vi "Blacklist Channel.vi"(8 "error in (no error)":errorcluster, 9 "Channel 2":string, 10 "Channel 1":string, 11 "SLSC Switch in":refnum<class "SLSC Switch.lvclass">) -> (0 "error out":errorcluster, 1 "New Entry?":bool, 3 "SLSC Switch out":refnum<class "SLSC Switch.lvclass">)   [LabVIEW 2015, in "SLSC Switch.lvclass"]
uses:
  SLSC Switch.lvclass
  SLSC Switch.lvclass/SLSC Switch.ctl
  Controls/Connection.ctl
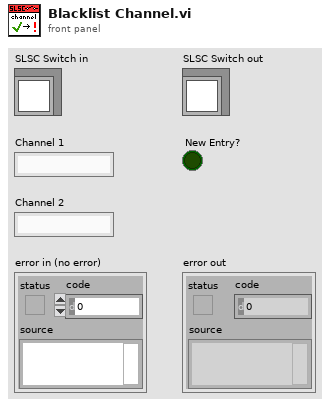
[diagram p1: front panel]
types:
  T1 = typedef "SLSC Switch.lvclass/Connection.ctl" = cluster{"channel 1":string, "channel 2":string}
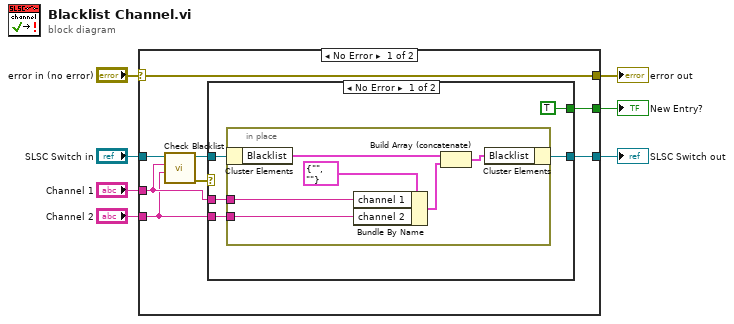
[diagram p0: block diagram]
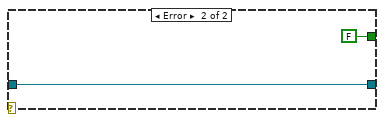
[diagram p2: hidden frame]
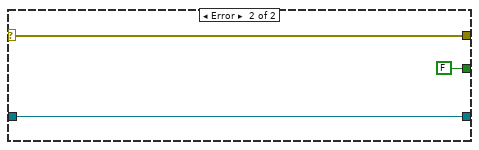
[diagram p3: hidden frame]
diagram:
  n1 = case shown="No Error" "error in (no error)" {
    selector: "error in (no error)" -> [w15 w31]
    tunnel: [w15 w31] -> w6
    tunnel: [w14 w30] -> w4
    tunnel: "SLSC Switch in" -> [w12 w30]
    tunnel: "Channel 1" -> [w11 _]
    tunnel: [w13 FALSE] -> w2
    tunnel: "Channel 2" -> [w10 _]
    frame No Error {
      n2 = call "Check Blacklist.vi"("Channel 2"=w10, "Channel 1"=w11, "SLSC Switch in"=w12) -> ("error out"=w9:errorcluster, "SLSC Switch out"=w8:refnum<class "SLSC Switch.lvclass">)  [unwired: 6 in, 1 out]
      n3 = case shown="No Error" w9 {
        tunnel: [w20 w28] -> w14
        tunnel: [TRUE FALSE] -> w13
        tunnel: w8 -> [w19 w28]
        tunnel: w11 -> [w18 _]
        tunnel: w10 -> [w17 _]
        frame No Error {
          n4 = in-place {
            in-place-border: w18 -> [w24]
            in-place-border: w17 -> [w23]
            n5 = in-place-cluster #1(w19) -> ("Blacklist"=w26:T1[])
            n6 = Bundle By Name(cluster=T1 {"channel 1"="", "channel 2"=""} ("connections"), "channel 1"=w24, "channel 2"=w23) -> (w22:T1)
            n7 = Build Array (concatenate)(w26, w22) -> (w21:T1[])
            n8 = in-place-cluster #1("Blacklist"=w21) -> (w20:refnum<class "SLSC Switch.lvclass">)
          }
        }
        frame Error {
        }
      }
    }
    frame Error {
    }
  }
  "error out" <- w6
  "SLSC Switch out" <- w4
  "New Entry?" <- w2
